vi "Update_Ch_Discription_client.vi"(1 "Channels to update In":T1[](array[typedef]) {"Duty" format="%016b"; "D" format="%#_5g"; "C" format="%#_5g"; "B" format="%#_5g"; "A" format="%#_5g"}) -> ()   [LabVIEW 2020]
doc: "This is an example of using features of the VI Server as a client. It shows how you might browse from one or more applications that may be exporting data from one or more data stations. \n\nThe example shows how to query a server for its list of exported VIs, how to get references to the VIs, and how call them with the Call By Reference function."
uses:
  Sub VIs/ADAM Controls/Ch_description_ADAM.ctl
  Sub VIs/ADAM Controls/Module_type_ADAM.ctl
  Sub VIs/ADAM Controls/Function_ADAM.ctl
  Sub VIs/ADAM Controls/Channel_State.ctl
  Sub VIs/ADAM Controls/Calib_type_ADAM.ctl
  Sub VIs/ADAM Controls/Address.ctl
  Anemometry/Anemometry Sub Vis/Controls/Global_mode.ctl
  Anemometry/Anemometry Sub Vis/Globals/Preference_global.vi
panel:
  in  "Server type":refnum<vi>
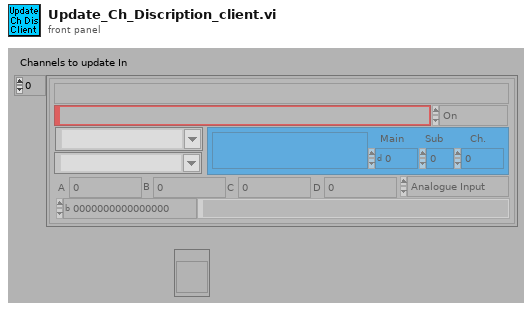
[diagram p1: front panel]
types:
  T1 = typedef "Ch_description_ADAM.ctl" = cluster{"Ch Name":string, "Type":T2, "Function":T3, "Ch State":T4, "Calibration type":T5, "A":dbl, "B":dbl, "C":dbl, "D":dbl, "Comments":string, "Address":T6, "String":string, "Duty":u16}
  T2 = typedef "Module_type_ADAM.ctl" = string
  T3 = typedef "Function_ADAM.ctl" = enum16{"Analogue Input", "Digital Input", "Event counter", "Event rate", "Analogue Output", "Digital Output", "Relay Output"}
  T4 = typedef "Channel_State.ctl" = enum16{"On", "Off", "Always On", "Always Off"}
  T5 = typedef "Calib_type_ADAM.ctl" = string
  T6 = typedef "Address.ctl" = cluster{"Main":i32, "Ch.":i32, "Sub":i32, "Port Name":string}
  T7 = typedef "Server_Comms.ctl" = enum16{"Do Not Link To Server", "Server Link Healthy"}
  T8 = enum16{"Append to Global", "Read Global then Clear"}
  T9 = typedef "Global_mode.ctl" = enum16{"Read Global", "Load Global From File", "Write Global to File"}
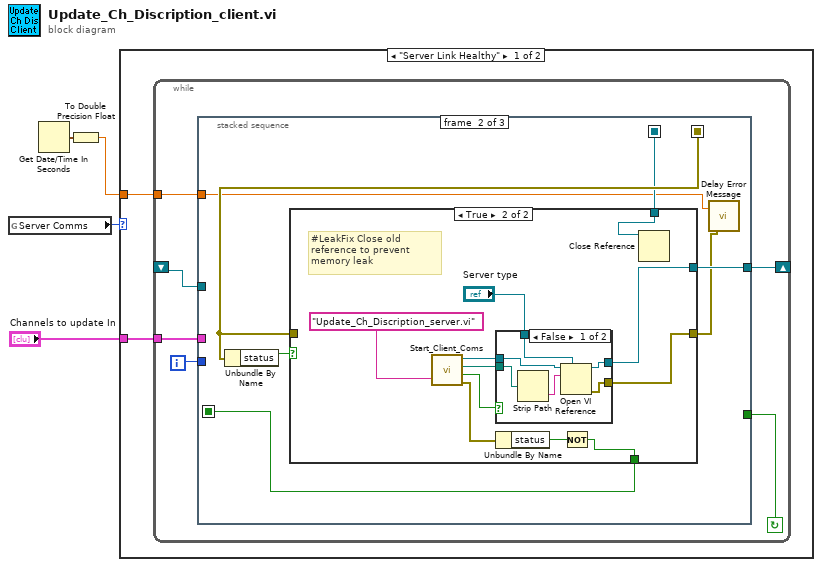
[diagram p0: block diagram]
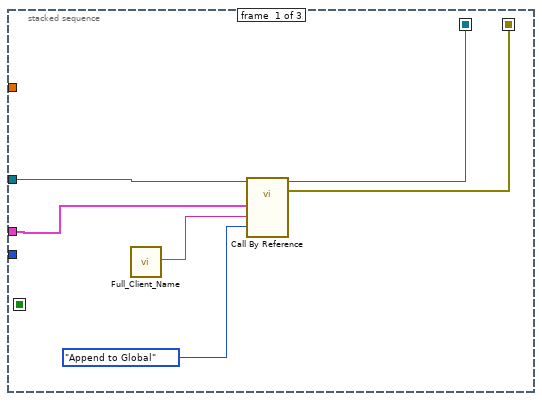
[diagram p2: hidden frame]
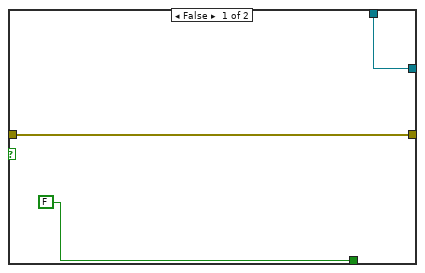
[diagram p3: hidden frame]
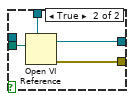
[diagram p4: hidden frame]
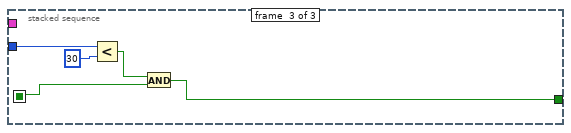
[diagram p5: hidden frame]
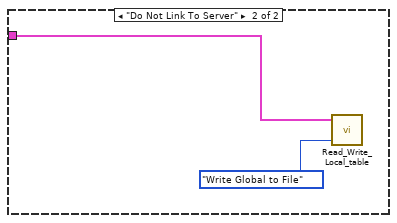
[diagram p6: hidden frame]
diagram:
  n1 = global read "Preference_global.vi" "Server Comms"() -> (w4:T7)
  n2 = Get Date/Time In Seconds() -> (seconds since 1Jan1904=w2:timestamp)
  n3 = To Double Precision Float(number=w2) -> (double precision float=w1:dbl)
  n4 = case shown="\"Server Link Healthy\"" w4 {
    tunnel: "Channels to update In" -> [w6 w55]
    tunnel: w1 -> [w5 _]
    frame "Server Link Healthy" {
      n5 = while {
        tunnel: w6 -> [w9]
        shift-left: _ -> [w12]
        shift-right: [w8] -> _
        tunnel: w5 -> [w7]
        i -> [w11]
        stop <- w10 continue-if-true
        n6 = stacked-sequence {
          seq-local: [w13 _ _] -> [_ w22 _]
          seq-local: [w18 _ _] -> [_ w23 _]
          seq-local: [_ w19 _] -> [_ _ w51]
          tunnel: w12 -> [w14 _ _]
          tunnel: [_ w25 _] -> w8
          tunnel: w11 -> [_ _ w52]
          tunnel: [_ _ w50] -> w10
          tunnel: w9 -> [w15 _ _]
          tunnel: w7 -> [_ w20 _]
          frame #0 {
            n7 = call "Full_Client_Name.vi"() -> ("Client Name"=w17:string)
            n8 = call-by-ref "?"(reference=w14, "Mode"=T8."Append to Global", "Client HD name"=w17, "Channels to update In"=w15) -> (reference out=w13:refnum<vi>, error out=w18:errorcluster)  [unwired: 1 in, 1 out]
          }
          frame #1 {
            n9 = Unbundle By Name(w23) -> ("status"=w24:bool)
            n10 = case shown="True" w24 {
              tunnel: [w27 w35] -> w25
              tunnel: w22 -> [w27 w32]
              tunnel: [w28 w33] -> w21
              tunnel: w23 -> [w28 _]
              tunnel: [FALSE w30] -> w19
              frame False {
              }
              frame True {
                # "#LeakFix Close old reference to prevent memory leak"
                n11 = call "Start_Client_Coms.vi"("VI name to run on server"="Update_Ch_Discription_server.vi") -> ("LabVIEW application reference"=w37:refnum<vi>, "Checked VI name"=w38:path, "Local Call"=w36:bool, "Error cluster"=w29:errorcluster)  [unwired: 1 in]
                n12 = case shown="False" w36 {
                  tunnel: [w44 w49] -> w35
                  tunnel: "Server type" -> [w42 w48]
                  tunnel: w38 -> [w41 w47]
                  tunnel: w37 -> [w40 _]
                  tunnel: [w43 w46] -> w33
                  frame False {
                    n13 = Strip Path(path=w41) -> (name=w45:string)  [unwired: 1 out]
                    n14 = Open VI Reference(type specifier VI Refnum (for type only)=w42, application reference (local)=w40, vi path=w45) -> (vi reference=w44:refnum<vi>, error out=w43:errorcluster)  [unwired: 1 in, 2 out]
                  }
                  frame True {
                    n15 = Open VI Reference(type specifier VI Refnum (for type only)=w48, vi path=w47) -> (vi reference=w49:refnum<vi>, error out=w46:errorcluster)  [unwired: 1 in, 3 out]
                  }
                }
                n16 = Unbundle By Name(w29) -> ("status"=w31:bool)
                n17 = Not(x=w31) -> (.not. x?=w30:bool)
                n18 = Close Reference(reference=w32) -> ()  [unwired: 1 in, 1 out]
              }
            }
            n19 = call "Delay Error Message.vi"("error in (no error)"=w21, "Seconds since 1904"=w20) -> ()  [unwired: 2 in]
          }
          frame #2 {
            n20 = Less?(x=w52, y=30) -> (x < y?=w54:bool)
            n21 = And(x=w54, y=w51) -> (x .and. y?=w50:bool)
          }
        }
      }
    }
    frame "Do Not Link To Server" {
      n22 = call "Read_Write_Local_table.vi"("Mode"=Global_mode."Write Global to File", "Channels Descriptions In"=w55) -> ()  [unwired: 1 in, 3 out]
    }
  }
